vi "StateMachineOperation.vi"() -> ()   [LabVIEW 2020]
panel:
  out "Shooter Eject":bool
  out "Right Ball Color":string
  out "Left Ball Color":string
  out "Opposite Color":string
  out "Ball Color":string
  out "Climber - Finished":bool
  out "Climber - Pull":bool
  out "Enable Shooter":bool
  # "Shooter"
  # "Conveyor"
  # "Climber"
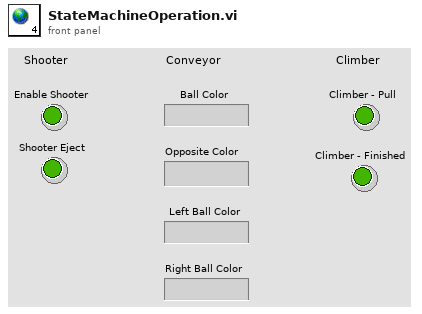
[diagram p1: front panel]
diagram:
